vi "Delete Category.vi"(8 "error in (no error)":errorcluster, 10 "Category":refnum<class "Category.lvclass">, 11 "Database in":refnum<class "Account History.lvclass">) -> (0 "error out":errorcluster, 3 "Database out":refnum<class "Account History.lvclass">)   [LabVIEW 2018, in "Account History.lvclass"]
uses:
  Account History.lvclass
  Category/Category.lvclass
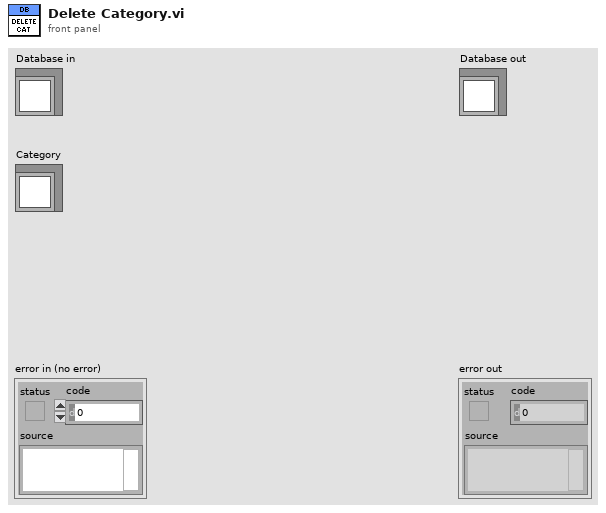
[diagram p1: front panel]
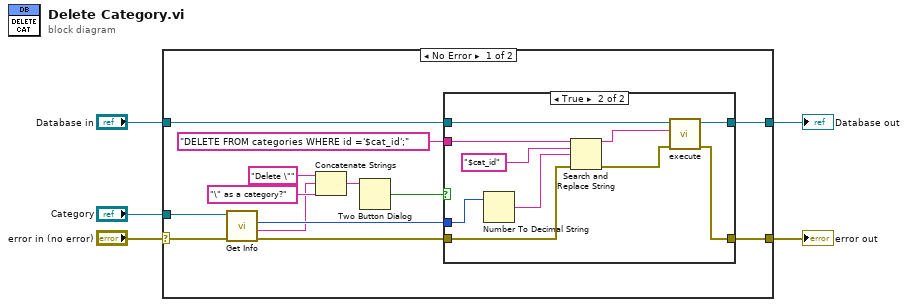
[diagram p0: block diagram]
diagram:
  n1 = case shown="No Error" "error in (no error)" {
    selector: "error in (no error)" -> [w6 w31]
    tunnel: "Database in" -> [w10 w32]
    tunnel: [w9 w32] -> w4
    tunnel: [w8 w31] -> w3
    tunnel: "Category" -> [w7 _]
    frame No Error {
      n2 = call "Get Info.vi"("error in (no error)"=w6, "Category in"=w7) -> ("error out"=w15:errorcluster, "Name"=w11:string, "id"=w12:i32)  [unwired: 6 in, 1 out]
      n3 = Concatenate Strings("Delete \"", w11, "\" as a category?" ("string")) -> (w16:string)
      n4 = Two Button Dialog(message=w16) -> (T button?=w14:bool)  [unwired: 2 in]
      n5 = case shown="True" w14 {
        tunnel: w10 -> [w20 w30]
        tunnel: [w20 w29] -> w9
        tunnel: w15 -> [w19 w23]
        tunnel: [w19 w27] -> w8
        tunnel: w12 -> [_ w28]
        tunnel: "DELETE FROM categories WHERE id ='$cat_id';" -> [_ w26]
        frame False {
        }
        frame True {
          n6 = Number To Decimal String(number=w28) -> (decimal integer string=w22:string)  [unwired: 1 in]
          n7 = Search and Replace String(input string=w26, search string="$cat_id", replace string=w22, error in=w23) -> (result string=w25:string, error out=w24:errorcluster)  [unwired: 4 in, 2 out]
          n8 = call "execute.vi"("error in (no error)"=w24, "SQL query"=w25, "Database in"=w30) -> ("error out"=w27:errorcluster, "Database out"=w29:refnum<class "Account History.lvclass">)  [unwired: 7 in]
        }
      }
    }
    frame Error {
    }
  }
  "error out" <- w3
  "Database out" <- w4
